vi "Periodic Tasks.vi"(8 "error in":errorcluster) -> ()   [LabVIEW 2014]
doc: "This VI runs in parallel to other tasks. It can contain as many user-defined periodic loops as you need. These can carry out PID or other sorts of timed response."
uses:
  ChassisLib/ChassisRefs.ctl
  <vilib>/Rock Robotics/WPI/Joystick/WPI_JoystickGetSetRefNum.vi
  ChassisLib/ChassisLib.lvlib
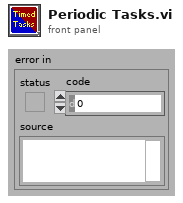
[diagram p1: front panel]
types:
  T1 = typedef "ChassisLib.lvlib/ChassisRefs.ctl" = enum16{"RobotDrive", "Compressor"}
  T2 = typedef "WPI_JoystickDevRef.ctl" = cluster{"Device":T3}
  T3 = typedef "WPI_JoystickDeviceEnum.ctl" = enum16{"USB 0", "USB 1", "USB 2", "USB 3", "USB 4", "USB 5"}
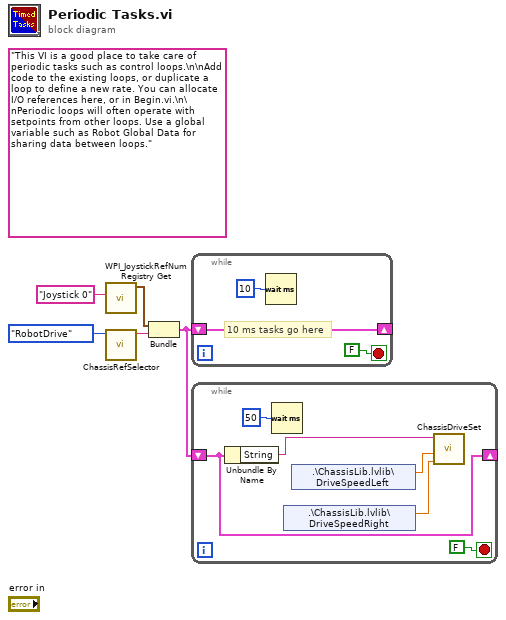
[diagram p0: block diagram]
diagram:
  (unwired) "This VI is a good place to take care of periodic tasks such as control loops.\n\nAdd code to the existing loops, or duplicate a loop to define a new rate. You can allocate I/O references here, or in Begin.vi.\n\nPeriodic loops will often operate with setpoints from other loops. Use a global variable such as Robot Global Data for sharing data between loops."
  n1 = call <vilib>:"WPI_JoystickRefNum Registry Get.vi"("refnum name"="Joystick 0") -> ("JoystickDevRef"=w4:T2)  [unwired: 1 in, 9 out]
  n2 = call "ChassisRefSelector.vi"("Enum 2"=ChassisRefs."RobotDrive") -> ("String"=w1:string)  [unwired: 10 in]
  n3 = Bundle("JoystickDevRef"=w4, "String"=w1) -> (w3:cluster{"JoystickDevRef":T2, "String":string})  [unwired: 1 out]
  n4 = while {
    shift-right: [w6] -> _
    shift-left: w3 -> [w6]
    stop <- FALSE stop-if-true
    # "10 ms tasks go here"
    n5 = Wait (ms)(milliseconds to wait=u32 10) -> ()  [unwired: 1 out]
  }
  n6 = while {
    shift-right: [w10] -> _
    shift-left: w3 -> [w10]
    stop <- FALSE stop-if-true
    n7 = Unbundle By Name(w10) -> ("String"=w9:string)
    n8 = Wait (ms)(milliseconds to wait=u32 50) -> ()  [unwired: 1 out]
    n9 = shared-variable ".\\ChassisLib.lvlib\\DriveSpeedRight"() -> (w11:dbl)  [unwired: 1 in, 1 out]
    n10 = shared-variable ".\\ChassisLib.lvlib\\DriveSpeedLeft"() -> (w12:dbl)  [unwired: 1 in, 1 out]
    n11 = call "ChassisDriveSet.vi"("Right axis value"=w11, "Left axis value"=w12, "DriveRef"=w9) -> ()  [unwired: 9 in]
  }
